vi "In Bounds 2D.vi"(0 "Top Left":T1 {"Axial Force" format="%.4f"; "Lateral Force" format="%.4f"}, 1 "Top Right":T1 {"Axial Force" format="%.4f"; "Lateral Force" format="%.4f"}, 2 "Bottom Right":T1 {"Axial Force" format="%.4f"; "Lateral Force" format="%.4f"}, 3 "Bottom Left":T1 {"Axial Force" format="%.4f"; "Lateral Force" format="%.4f"}, 4 "Lateral":dbl, 5 "Axial":dbl) -> (14 "InBounds":bool)   [LabVIEW 2016, in "Test Actuator State.lvclass"]
uses:
  Test Actuator State.lvclass
  Typedefs/ForcePair.ctl
  Typedefs/FAMT Typedefs.lvlib
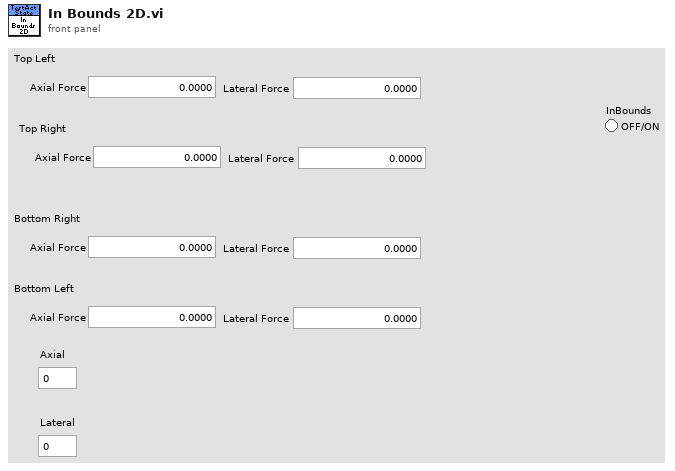
[diagram p1: front panel]
types:
  T1 = typedef "FAMT Typedefs.lvlib/ForcePair.ctl" = cluster{"Axial Force":dbl, "Lateral Force":dbl}
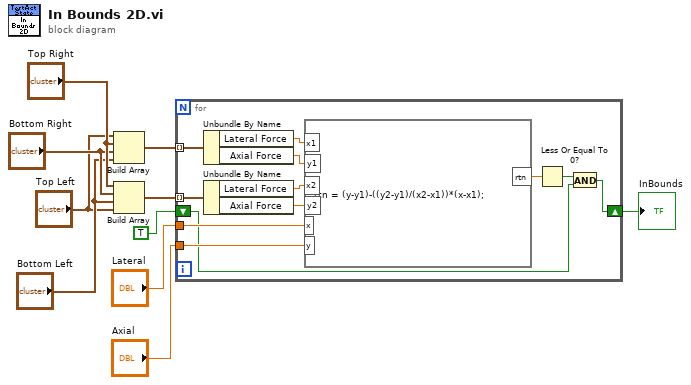
[diagram p0: block diagram]
diagram:
  n1 = Build Array("Top Left", "Top Right", "Bottom Right", "Bottom Left") -> (w6:T1[])
  n2 = Build Array("Top Right", "Bottom Right", "Bottom Left", "Top Left") -> (w5:T1[])
  n3 = for {
    tunnel: w6 -> [w22] mode=indexing
    tunnel: w5 -> [w21] mode=indexing
    tunnel: "Lateral" -> [w16]
    tunnel: "Axial" -> [w15]
    shift-right: [w12] -> w1
    shift-left: TRUE -> [w11]
    n4 = Unbundle By Name(w22) -> ("Lateral Force"=w20:dbl, "Axial Force"=w19:dbl)
    n5 = Unbundle By Name(w21) -> ("Lateral Force"=w18:dbl, "Axial Force"=w17:dbl)
    n6 = formula code="rtn = (y-y1)-((y2-y1)/(x2-x1))*(x-x1);"("x1"=w20, "y1"=w19, "x2"=w18, "y2"=w17, "x"=w16, "y"=w15) -> ("rtn"=w14:dbl)
    n7 = Less Or Equal To 0?(x=w14) -> (x <= 0?=w13:bool)
    n8 = And(x=w13, y=w11) -> (x .and. y?=w12:bool)
  }
  "InBounds" <- w1
